vi "AssertMultiChannelLoopbackForMappedChannels.vi"(4 "Tolerance (0.01)":dbl=0.01 format="%#_13g", 6 "output values":dbl[](array[numeric]), 7 "Timeout (1 second)":dbl=0.1 format="%#_13g", 8 "error in (no error)":errorcluster, 10 "output channels and mapped input channels":T1(array[cluster]), 11 "VeriStand Test Case in":refnum<class "VeriStandTestCase.lvclass">) -> (0 "error out":errorcluster, 3 "VeriStand Test Case out":refnum<class "VeriStandTestCase.lvclass">)   [LabVIEW 2027, in "VeriStandTestCase.lvclass"]
uses:
  VeriStandTestCase.lvclass
  VeriStandTestCase.lvclass/VeriStandTestCase.ctl
  <vilib>/NI VeriStand/Execution/Workspace/NI VeriStand - Set Multiple Channel Values.vi
  <vilib>/NI VeriStand/Execution/Workspace/NI_VS Workspace ExecutionAPI.lvlib
  VeriStandTestUtilities/VeriStandTestUtilities.lvlib
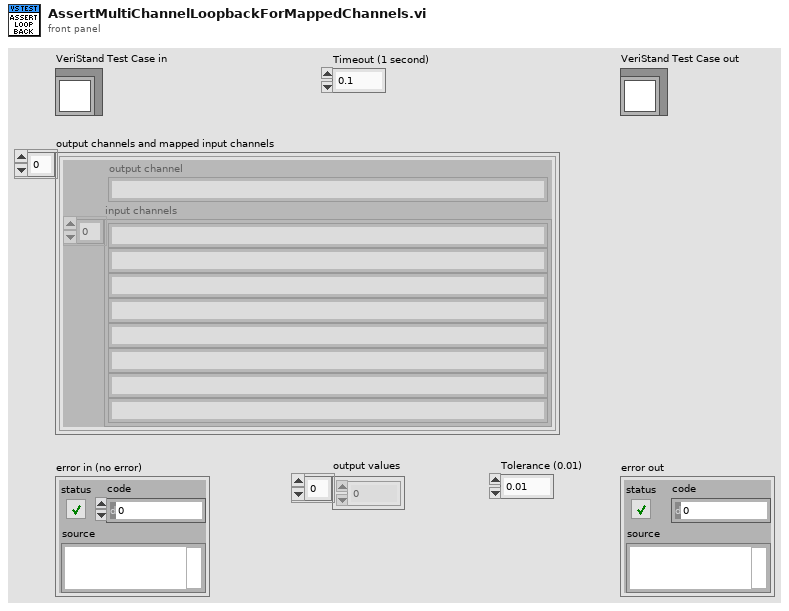
[diagram p1: front panel]
types:
  T1 = cluster{"output channel":string, "input channels":string[]}[]
  T2 = typedef "NI_VS Workspace ExecutionAPI.lvlib/WorkspaceAPI.ctl" = refnum<k39>
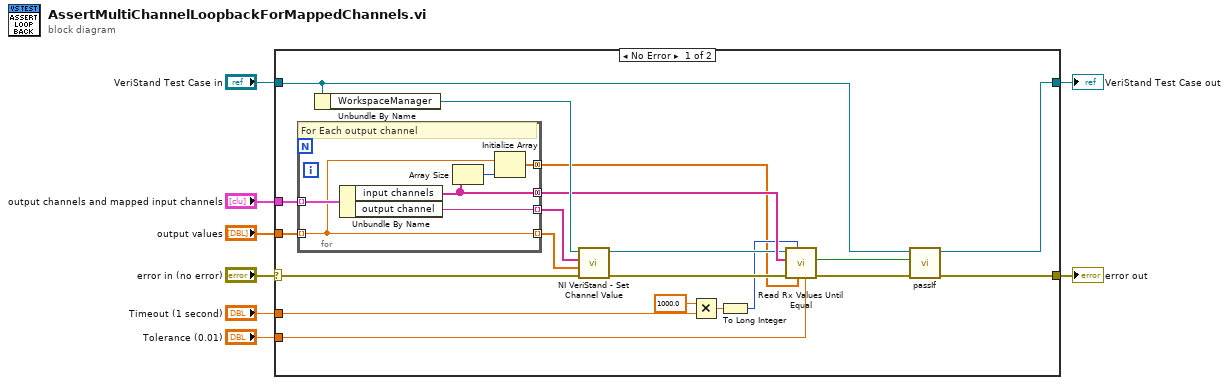
[diagram p0: block diagram]
diagram:
  n1 = case shown="No Error" "error in (no error)" {
    selector: "error in (no error)" -> [w28 w35]
    tunnel: [w18 w35] -> w8
    tunnel: "output channels and mapped input channels" -> [w26 _]
    tunnel: "output values" -> [w23 _]
    tunnel: "Timeout (1 second)" -> [w13 _]
    tunnel: "Tolerance (0.01)" -> [w14 _]
    tunnel: "VeriStand Test Case in" -> [w17 w36]
    tunnel: [w19 w36] -> w3
    frame No Error {
      n2 = for {
        tunnel: w26 -> [w34] mode=indexing
        tunnel: [w30] -> w25 mode=indexing
        tunnel: [w29] -> w24 mode=indexing
        tunnel: w23 -> [w29] mode=indexing
        tunnel: [w32] -> w9 mode=concatenating
        tunnel: [w31] -> w22 mode=concatenating
        # "For Each output channel"
        n3 = Unbundle By Name(w34) -> ("input channels"=w31:string[], "output channel"=w30:string)
        n4 = Array Size(array=w31) -> (size(s)=w33:i32)
        n5 = Initialize Array(w29, w33) -> (w32:dbl[])
      }
      n6 = Unbundle By Name(w17) -> ("WorkspaceManager"=w27:T2)
      n7 = call-poly <vilib>:"NI VeriStand - Set Channel Value.vi"("error in (no error)"=w28, "Values"=w24, "Channels"=w25, "WorkspaceManager in"=w27) -> ("error out"=w16:errorcluster, "WorkspaceManager out"=w21:T2)  [unwired: 6 in]
      n8 = Multiply(x=1000.0, y=w13) -> (x*y=w11:dbl)
      n9 = To Long Integer(number=w11) -> (32bit integer=w10:i32)
      n10 = call "Read Rx Values Until Equal.vi"("tolerance (0.01)"=w14, "expected values"=w9, "timeout (1000 ms)"=w10, "error in"=w16, "Rx aliases"=w22, "workspace manager in"=w21) -> ("error out"=w20:errorcluster, "values equal expected"=w15:bool)  [unwired: 3 in, 1 out]
      n11 = call-dynamic "passIf.vi"("error in (no error)"=w20, "pass"=w15, "TestCase in"=w17) -> ("error out"=w18:errorcluster, "TestCase out"=w19:refnum<class "VeriStandTestCase.lvclass">)  [unwired: 7 in]
    }
    frame Error {
    }
  }
  "error out" <- w8
  "VeriStand Test Case out" <- w3
